vi "correccion2.vi"(9 "orden 2":T1(array[ring]), 10 "opciones":bool[](array[boolean])) -> (2 "orden":T1(array[ring]))   [LabVIEW 2016]
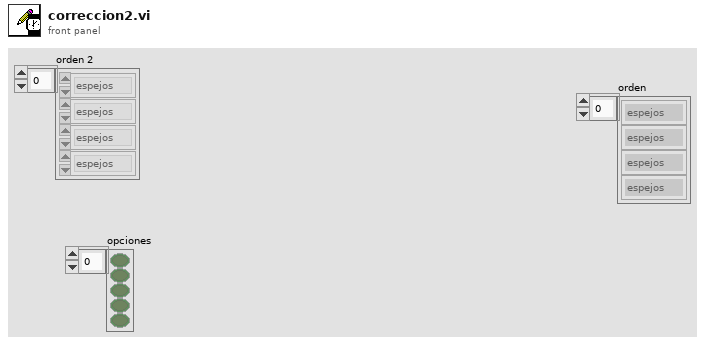
[diagram p1: front panel]
types:
  T1 = enum16{"espejos", "polarizador", "voltaje", "potenciometro y lockin", "CCD"}[]
  T2 = enum16{"espejos", "polarizador", "voltaje", "potenciometro y lockin", "CCD"}
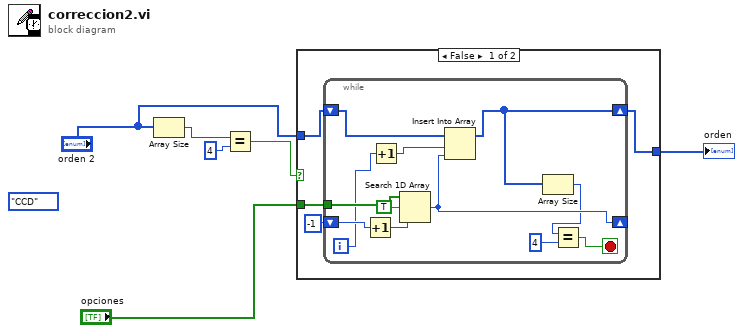
[diagram p0: block diagram]
diagram:
  (unwired) T2."CCD" ("Enum")
  n1 = Array Size(array="orden 2") -> (size(s)=w6:i32)
  n2 = Equal?(x=w6, y=4) -> (x = y?=w4:bool)
  n3 = case shown="False" w4 {
    tunnel: [w7 w23] -> w3
    tunnel: "orden 2" -> [w8 w23]
    tunnel: "opciones" -> [w10 _]
    frame False {
      n4 = while {
        tunnel: w10 -> [w22]
        shift-right: [w20] -> _
        shift-left: -1 -> [w19]
        shift-right: [w16] -> w7
        shift-left: w8 -> [w17]
        i -> [w11]
        stop <- w15 stop-if-true
        n5 = Increment(x=w19) -> (x+1=w18:i32)
        n6 = Increment(x=w11) -> (x+1=w12:i32)
        n7 = Search 1D Array(1D array=w22, element=TRUE, start index (0)=w18) -> (index of element=w20:i32)
        n8 = Insert Into Array(array=w17, index=w12, new element=w20) -> (w16:T1)
        n9 = Array Size(array=w16) -> (size(s)=w14:i32)
        n10 = Equal?(x=w14, y=4) -> (x = y?=w15:bool)
      }
    }
    frame True {
    }
  }
  "orden" <- w3
